vi "ErrorHandling.generalErrorHanlderInclObjRef.vi"(6 "LastCommand(optional)":string, 8 "error in":errorcluster, 9 "StopOnError":bool, 10 "Comment(optional)":string, 11 "ErrorHandling(optional)":refnum<data-value>) -> (0 "error out":errorcluster, 2 "Stop":bool, 3 "ErrorHandling out":refnum<data-value>)   [LabVIEW 2016, in "ErrorHandling.lvclass"]
doc: "Generelle Error Handling Methode, kann direkt so eingesetzt werden\n\n17.04.17 / sige"
uses:
  ErrorHandling.lvclass
  ErrorHandling.lvclass/ErrorHandling.ctl
  <vilib>/Utility/error.llb/Clear Errors.vi
  Package Libraries/StringFunctions/StringFunctions_ReplaceAllBlindSigns.vi
  Package Libraries/Message Queue/MessageQueue_GetQueue.vi
  Package Libraries/Message Queue/MessageQueue_EnqueueElement.vi
  Package Libraries/Message Queue/MessageQueue_DequeueElement.vi
  <vilib>/dlg_ctls.llb/Space Constant.vi
  ErrorHandling.addLastErrorToFile.vi
  <vilib>/Utility/error.llb/Search and Replace Pattern.vi
  <vilib>/Utility/error.llb/Trim Whitespace.vi
  Package Libraries/TimingFunctions/TimingFunctions_getUtcTimestamp.vi
  Package Libraries/Message Queue/MessageQueue_ReleaseQueue.vi
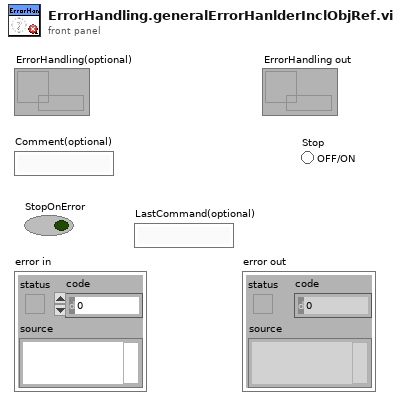
[diagram p1: front panel]
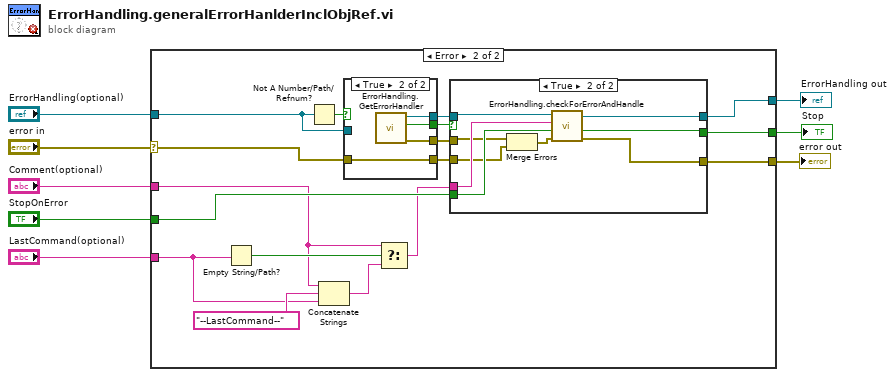
[diagram p0: block diagram]
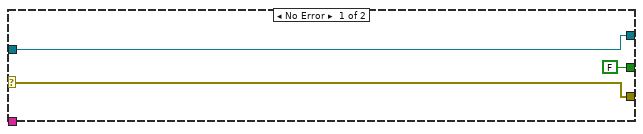
[diagram p2: hidden frame]
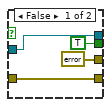
[diagram p3: hidden frame]
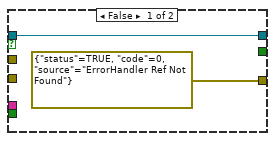
[diagram p4: hidden frame]
diagram:
  n1 = case shown="Error" "error in" {
    selector: "error in" -> [w9 w12]
    tunnel: [w9 w28] -> w8
    tunnel: [w11 w27] -> w7
    tunnel: "ErrorHandling(optional)" -> [w11 w26]
    tunnel: [FALSE ("Stop") w25] -> w5
    tunnel: "StopOnError" -> [_ w24]
    tunnel: "Comment(optional)" -> [_ w15]
    tunnel: "LastCommand(optional)" -> [_ w14]
    frame No Error {
    }
    frame Error {
      n2 = Empty String/Path?(string/path=w14) -> (empty?=w18:bool)
      n3 = Not A Number/Path/Refnum?(number/path/refnum=w26) -> (NaN/Path/Refnum?=w20:bool)
      n4 = Concatenate Strings(w15, "--LastCommand--" ("string"), w14) -> (w13:string)
      n5 = case shown="True" w20 {
        tunnel: [w32 w35] -> w23
        tunnel: [TRUE ("Found?") w34] -> w22
        tunnel: [errorcluster {"status"=FALSE, "code"=0, "source"=""} ("ErrorOut") w36] -> w21
        tunnel: w26 -> [w32 _]
        tunnel: w12 -> [w30 w33]
        tunnel: [w30 w33] -> w19
        frame False {
        }
        frame True {
          n6 = call "ErrorHandling.GetErrorHandler.vi"() -> ("ErrorOut"=w36:errorcluster, "Found?"=w34:bool, "ErrorRef"=w35:refnum<data-value>)  [unwired: 9 in]
        }
      }
      n7 = Select(t=w15, s=w18, f=w13) -> (s? t:f=w17:string)
      n8 = case shown="True" w22 {
        tunnel: [errorcluster {"status"=TRUE, "code"=0, "source"="ErrorHandler Ref Not Found"} ("error IO") w45] -> w28
        tunnel: w23 -> [w37 w47]
        tunnel: w21 -> [_ w41]
        tunnel: [w37 w44] -> w27
        tunnel: w17 -> [_ w46]
        tunnel: [_ w43] -> w25
        tunnel: w24 -> [_ w42]
        tunnel: w19 -> [_ w39]
        frame False {
        }
        frame True {
          n9 = Merge Errors(w41, w39) -> (w40:errorcluster)
          n10 = call "ErrorHandling.checkForErrorAndHandle.vi"("error in (no error)"=w40, "StopOnError"=w42, "Comment"=w46, "ErrorHandling in"=w47) -> ("error out"=w45:errorcluster, "Stop"=w43:bool, "ErrorHandling out"=w44:refnum<data-value>)  [unwired: 5 in]
        }
      }
    }
  }
  "Stop" <- w5
  "ErrorHandling out" <- w7
  "error out" <- w8
